vi "SubPanel_DataCollection_Rev11_v17.vi"(0 "DCPowerInformationClusterArray_Input":T8(array[cluster]), 1 "VISAPowerInfoInputArray":T5(array[cluster]), 2 "Run Data SubPanel Input":T4, 3 "RF Block Input Array":T3[](array[typedef]), 4 "Oscilloscope Info Array":T7(array[cluster]) {"vertical coupling" items=["AC", "DC", "Ground"]}, 5 "Plot Color Array":u32[](array[colorbox])=[16711686, 65351, 8978420, 14474240, 16139007, 16752640, 8958719, 16758973, 16777215, 46792, 11992992, 12961221, 16763690, 12600063, 16711835, 2953983, 40796, 13111296, 13352613, 9221011, 12964076, 12819897, 65442, 16776704, 14540253, 16740729, 10658047, 10813344, 16753521, 13413843, 8691115, 10339240, 14401205, 16746704, 7467519, 16775978, 13872558, 11387603, 13354405, 10420227, 13107364, 4060, 35208, 11817216, 7566080, 40796, 7539456, 2837073, 6372186, 7499083, 10648702, 16757152], 6 "New Run?":bool, 7 "error in":errorcluster) -> (20 "DCPowerInformationClusterArray_Output":T8(array[cluster]), 21 "VISAPowerInfoInputOutput":T5(array[cluster]), 22 "Run Data SubPanel Output":T4, 23 "RF Subpanel Output":T3[](array[typedef]), 24 "Oscilloscope Info Array":T7(array[cluster]) {"vertical coupling" items=["AC", "DC", "Ground"]}, 25 "Reinitialize?":bool, 26 "Data Was Collected?":bool, 27 "error out":errorcluster)   [LabVIEW 2019]
uses:
  Controls/DataBlockControl.ctl
  <instrlib>/niScope/Controls/niScope vertical coupling.ctl
  Controls/RFBlockControl.ctl
  Controls/QueueDataControl_V3.ctl
  <instrlib>/niScope/Acquire/Fetch/niScope Multi Fetch Binary 16.vi
  <vilib>/Utility/file.llb/Write Delimited Spreadsheet (string).vi
panel:
  in  "stop":bool
  out "wfm 2":i16[][][](array[numeric])
  out "Array":i32[](array[numeric])
  out "wfm":i16[][](array[numeric])
  in  "Total Time X Min":dbl
  in  "Total Time X Max":dbl
  in  "Total Current Y Min":dbl
  in  "Total Current Y Max":dbl
  in  "Total Voltage Y Min":dbl
  in  "Total Voltage Y Max":dbl
  in  "Total Measurement Range Update":bool
  in  "Device Powered?":bool=TRUE
  out "output cluster":T2 {"vertical coupling" items=["AC", "DC", "Ground"]}
  in  "Live Measurement Range Update":bool
  in  "Live Current Y Min":dbl
  in  "Live Current Y Max":dbl
  in  "Live Voltage Y Min":dbl
  in  "Live Voltage Y Max":dbl
  out "Current Measurements Live":cluster{dbl[], dbl[]}[](graph)
  out "Voltage Measurements Live":cluster{dbl[], dbl[]}[](graph)
  out "Voltage Waveform Array":waveform(dbl)[](graph)
  out "Current Waveform Array":waveform(dbl)[](graph)
  out "Current Measurements Total":cluster{dbl[], dbl[]}[](graph)
  out "Voltage Measurements Total":cluster{dbl[], dbl[]}[](graph)
  out "Exiting":bool
  out "Full Run Information":string
  out "Ready For Next Run?":bool
  in  "Next Run":bool
  out "Recording Data":bool
  in  "Record Data Toggle":bool
  out "error of collection":errorcluster
  in  "force exit SubVI":bool
  out "RF Block Parameters Output":T3
  in  "Oscilloscope Info Array":T6(array[cluster]) {"vertical coupling" items=["AC", "DC", "Ground"]}
  out "seconds since 1Jan1904 2":timestamp
  out "seconds since 1Jan1904":timestamp
  out "Numeric 2":i32
  out "Numeric":i32
  out "RFSourceInfoArray":string[][](array[string])
  out "OscilloscopeInfoArray":string[][](array[string])
  out "DCPowerInfoArray":string[][](array[string])
  # "Background information (Important)\nThere are three sets of voltage/current graphs\n\nOne is live always and just shows what all the channels look like _______ Waveform Array\n\nOne is live when measuring and shows some duration of the recording _______ Measurements Live\n\nOne shows the entire duration of the run, but it will take a few seconds to compile, just be patient it will populate\n\n\nInstructions (More Important)"
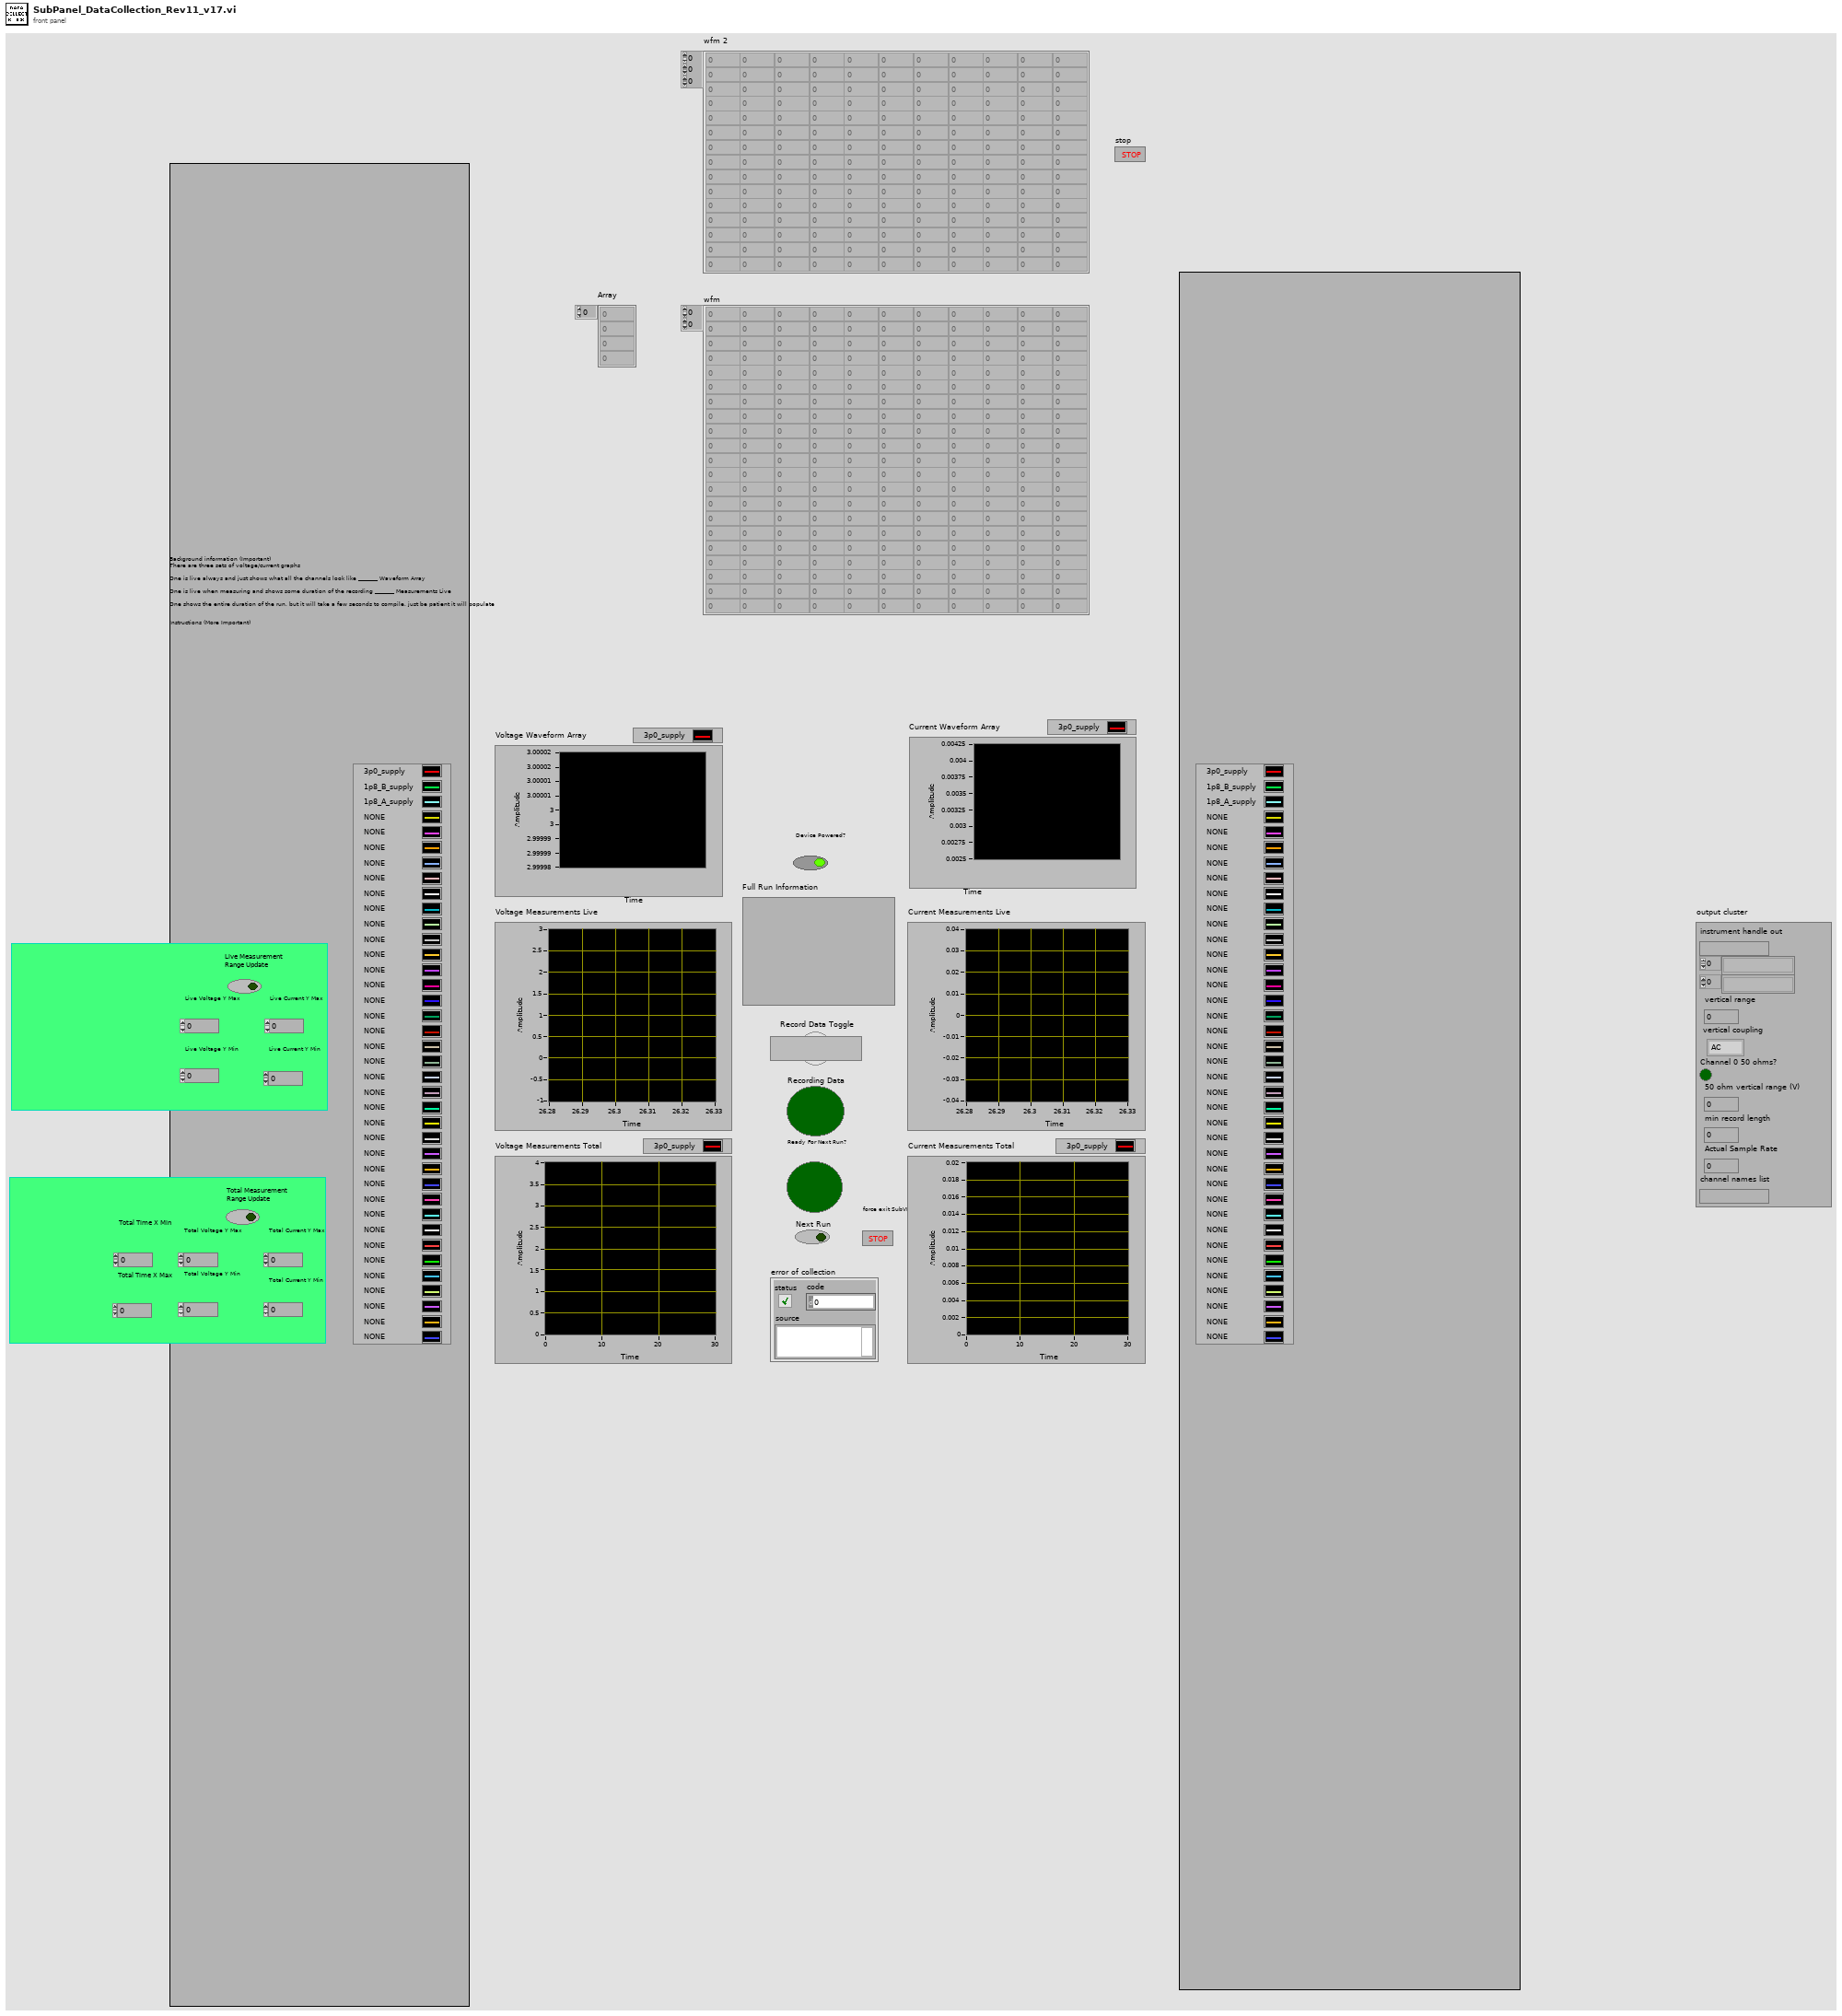
[diagram p1: front panel]
types:
  T1 = typedef "niScope vertical coupling.ctl" = i32
  T2 = cluster{"instrument handle out":refnum<k15>, string[], string[], "vertical range":dbl, "vertical coupling":T1, "Channel 0 50 ohms?":bool, "50 ohm vertical range (V)":dbl, "min record length":i32, "Actual Sample Rate":dbl, "channel names list":string}
  T3 = typedef "RFBlockControl.ctl" = cluster{"VISA resource name":refnum<visa-resource-name>, "RF Power State In":bool, "Frequency (GHz) Output":dbl, "Power (dBm) Output":dbl, "Instrument Name":string}
  T4 = typedef "DataBlockControl.ctl" = cluster{"Run Folder Parent Directory":path, "DUT":string, "Ion (ex Kr)":string, "Board Number":string, "Effective LET":string, "Test Type":enum16{"Single Event Latchup", "Single Event Transient", "Single Event Upset"}}
  T5 = cluster{"VISA resource name":refnum<visa-resource-name>, "String List":string, string[], "Input Array (Voltage,Current_Limit)":dbl[], "Input Array (Voltage,Current_Limit)":dbl[], "Channel Names":string[], "read buffer":string}[]
  T6 = cluster{"instrument handle out":refnum<k15>, "channel numbers array":string[], "channel names array":string[], "vertical range":dbl, "vertical coupling":T1, "Channel 0 50 ohms?":bool, "50 ohm vertical range (V)":dbl, "min record length":i32, "Actual Sample Rate":dbl}[]
  T7 = cluster{"instrument handle out":refnum<k15>, string[], string[], "vertical range":dbl, "vertical coupling":T1, "Channel 0 50 ohms?":bool, "50 ohm vertical range (V)":dbl, "min record length":i32, "Actual Sample Rate":dbl, "channel names list":string}[]
  T8 = cluster{"IVI Refnum out":refnum<k15>, "Active Channel Numbers String List":string, "Active Channel Numbers Array":string[], "Active Channel Voltage Array":dbl[], "Active Channel Names Array":string[], "Active Channel Current Limit Array":dbl[], "Active Channel Measure Record Delta Time Array":dbl[], "All Channel Numbers Array":string[]}[]
  T9 = typedef "QueueDataControl_V3.ctl" = cluster{"Array of fetched data":dbl[][][], "Channel Names Array":string[], "Voltage Waveform Array":waveform(dbl)[], "Current Waveform Array":waveform(dbl)[], "Resetting Time":timestamp}
  T10 = cluster{"IVI Refnum out":refnum<k15>, string, "voltage level channel 23":dbl, "Channel Name 23":string, "Current Limit":dbl, "Measure Record dt":dbl, string}[]
  T11 = cluster{timestamp[], "wfm info":cluster{"actualSamples":i32, "absoluteInitialX":dbl, "relativeInitialX":dbl, "xIncrement":dbl, "offset":dbl, "gain":dbl, "reserved1":dbl, "reserved2":dbl}[][], "wfm":i16[][][]}
  T12 = cluster{"actualSamples":i32, "absoluteInitialX":dbl, "relativeInitialX":dbl, "xIncrement":dbl, "offset":dbl, "gain":dbl, "reserved1":dbl, "reserved2":dbl}[]
  T13 = cluster{"created path":path, "DCPowerInformation_byChannel":cluster{"IVI Refnum out":refnum<k15>, string, "voltage level channel 23":dbl, "Channel Name 23":string, "Current Limit":dbl, "Measure Record dt":dbl, string}[], string[]}
  T14 = cluster{"Array of fetched data":dbl[][], string, i32[]}
  T15 = enum16{"open", "replace", "create", "open or create", "replace or create", "replace or create with confirmation"}
  T16 = enum16{"Single Event Latchup", "Single Event Transient", "Single Event Upset"}
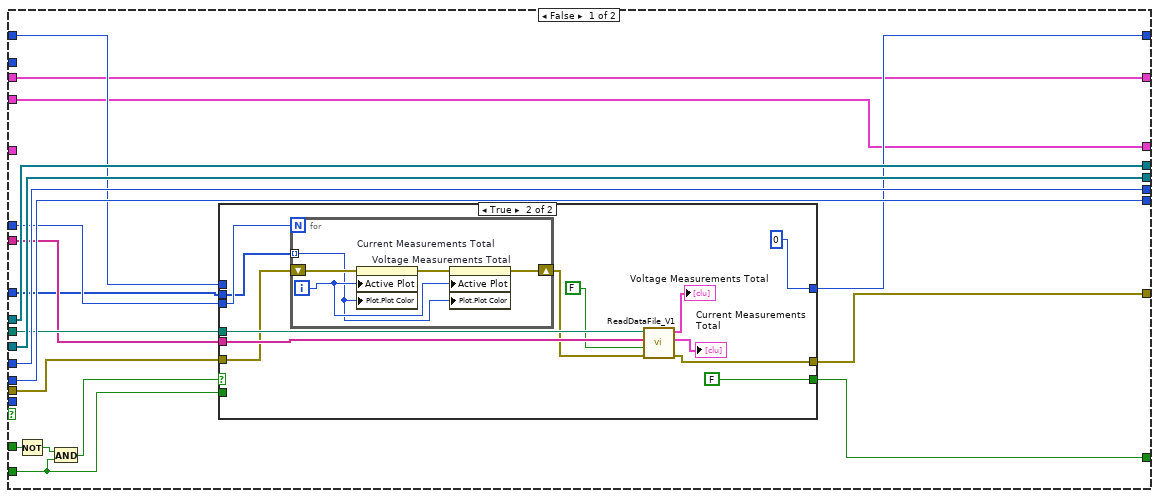
[diagram p7: hidden frame]
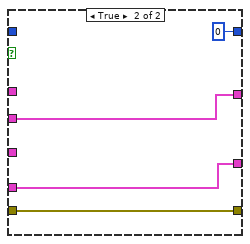
[diagram p9: hidden frame]
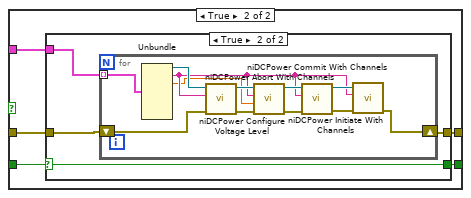
[diagram p10: hidden frame]
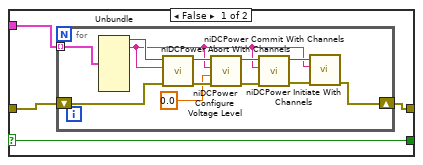
[diagram p11: hidden frame]
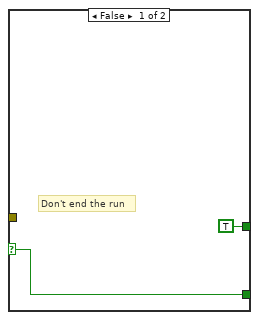
[diagram p12: hidden frame]
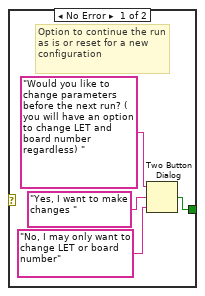
[diagram p13: hidden frame]
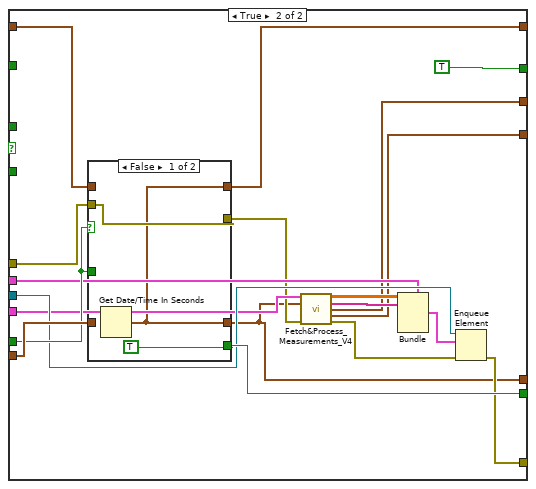
[diagram p16: hidden frame]
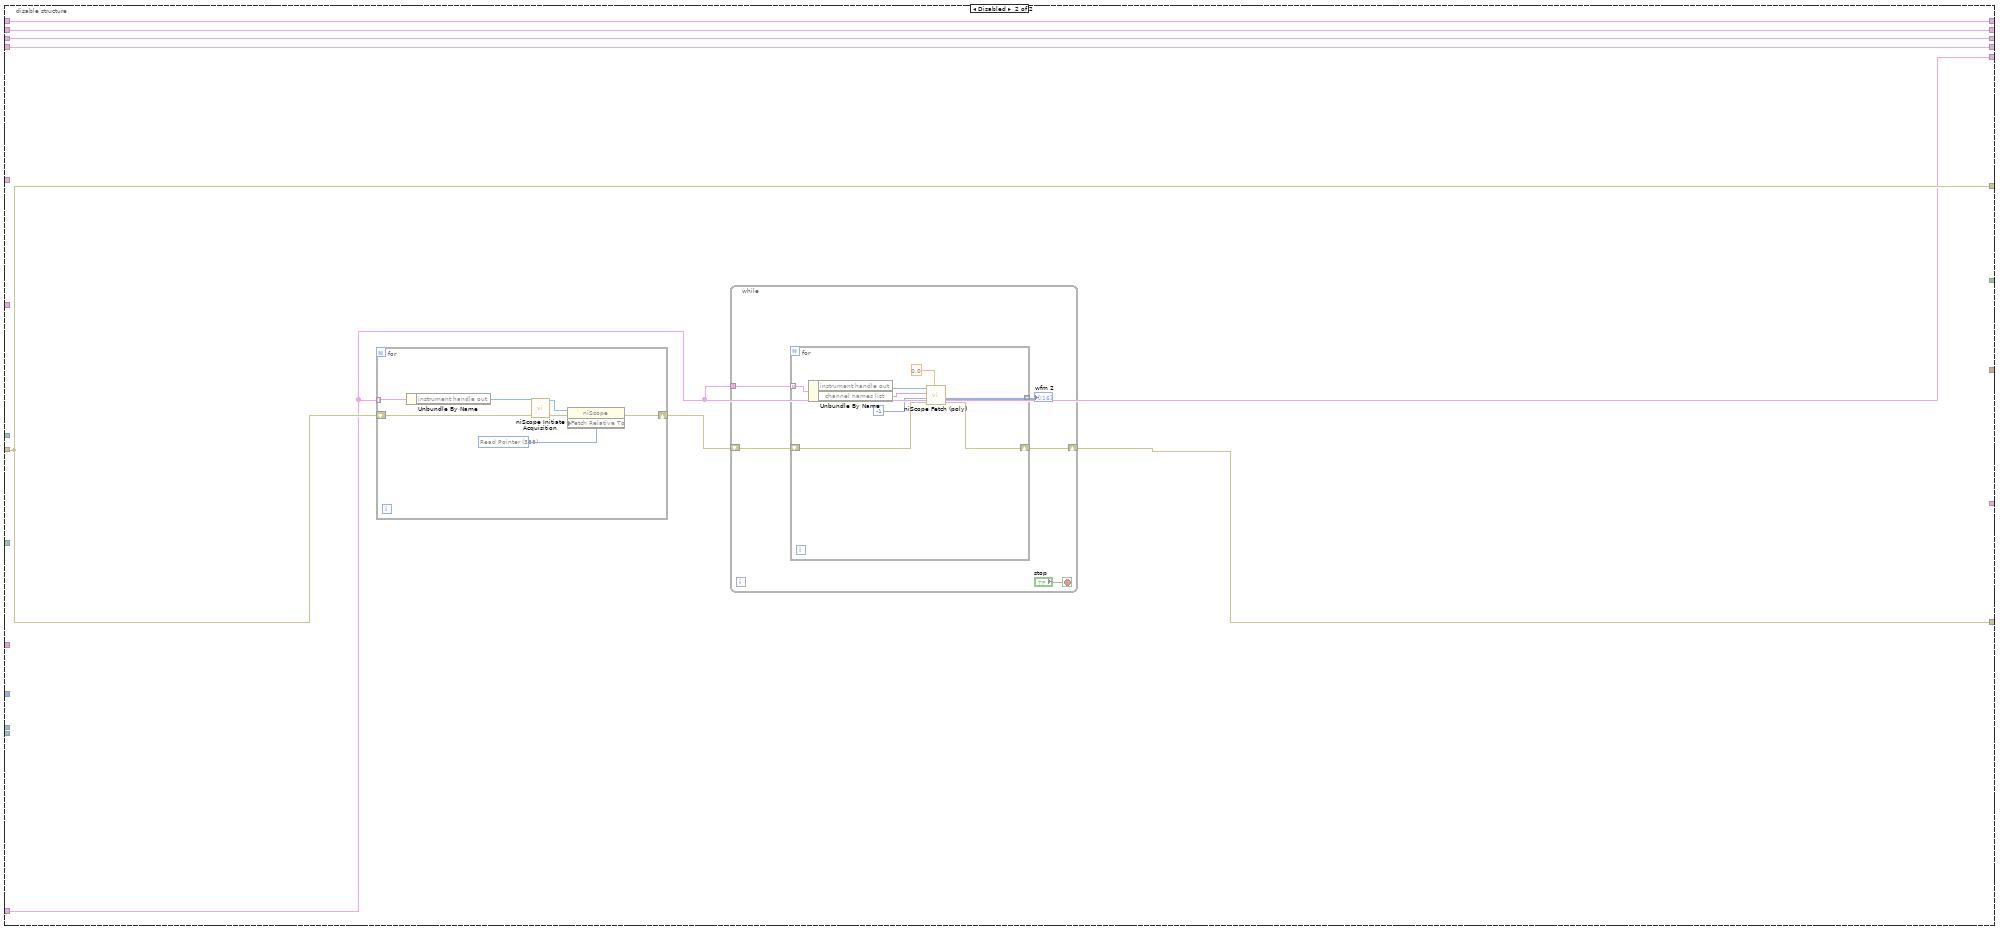
[diagram p18: hidden frame]
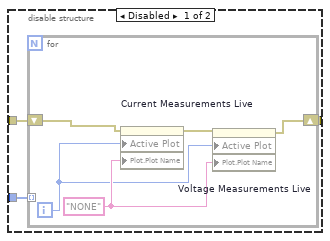
[diagram p19: hidden frame]
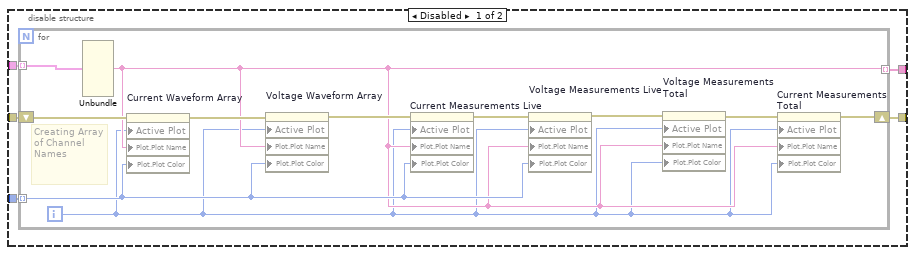
[diagram p20: hidden frame]
diagram:
  (unwired) string[] ["Instrument Name", "Channel Name", "Instrument Channel Number", "Voltage (V)", "Current Limit (A)", "Measure Record delta Time (s)"] ("new element/subarray")
  w41 = T9 {"Array of fetched data"=[], "Channel Names Array"=[], "Voltage Waveform Array"=[], "Current Waveform Array"=[], "Resetting Time"=timestamp(0 s since 1904-01-01)} ("DCPower Queue Data Double Array Format")
  (unwired) T9 {"Array of fetched data"=[], "Channel Names Array"=[], "Voltage Waveform Array"=[], "Current Waveform Array"=[], "Resetting Time"=timestamp(0 s since 1904-01-01)} ("DCPower Double Array Queue")
  (unwired) T4 {"Run Folder Parent Directory"=path "", "DUT"="", "Ion (ex Kr)"="", "Board Number"="", "Effective LET"="", "Test Type"=enum."Single Event Latchup"} ("Run Data Configuration")
  # "Initiating the queue"
  # "echoing run information"
  # "Checking if this is a new run. If it is, a new folder is created along with references to a datafile node. If it is not new (i.e. you didn't start recording data because you needed to make a last minute change and pressed forced exit subvi), the previous folder that is theoretically empty (or just has the .txt files is used"
  # "If yes, you go into this subVI"
  # "This is the message at the beginning confirming if you want to make small changes to the program (i.e. LET)"
  # "Parameters from the configuration stage of this program"
  # "Need to change to reflect number of channels that are being recorded. Collect this from a parameters file eventually that will be created"
  # "Initiating all of the DC Power instruments (doing this here so because we force abort channels in the DCPower setup because buffer overflow issues. Iterating over the instrument array and the active channel list"
  n1 = flat-sequence {
    tunnel: [w74] -> w55
    tunnel: "error in" -> [w64]
    tunnel: [w78] -> w59
    tunnel: "Run Data SubPanel Input" -> [w66]
    frame #0 {
      n2 = disable-structure shown="Enabled" {
        disable-tunnel: w64 -> [w81 w92]
        disable-tunnel: [w90 w92] -> w63
        frame Enabled {
          n3 = property on="Voltage Measurements Live" class="XYGraph (strict)"(error in=w81, "BG Color"=u32 0 ("Plot.Plot Color"), "Plot.Plot Interpolation"=u8 2) -> (error out=w80:errorcluster)  [unwired: 1 in, 1 out]
          n4 = property on="Current Measurements Live" class="XYGraph (strict)"(error in=w80, "BG Color"=u32 0 ("Plot.Plot Color"), "Plot.Plot Interpolation"=u8 2) -> (error out=w79:errorcluster)  [unwired: 1 in, 1 out]
          n5 = property on="Voltage Measurements Total" class="XYGraph (strict)"(error in=w79, "BG Color"=u32 0 ("Plot.Plot Color"), "Plot.Plot Interpolation"=u8 2) -> (error out=w91:errorcluster)  [unwired: 1 in, 1 out]
          n6 = property on="Current Measurements Total" class="XYGraph (strict)"(error in=w91, "BG Color"=u32 0 ("Plot.Plot Color"), "Plot.Plot Interpolation"=u8 2) -> (error out=w90:errorcluster)  [unwired: 1 in, 1 out]
        }
        frame Disabled {
        }
      }
      n7 = local write "Voltage Measurements Total"(cluster{dbl[], dbl[]}[] [] ("Voltage Measurements")) -> ()
      n8 = local write "Current Measurements Total"(cluster{dbl[], dbl[]}[] [] ("Current Measurements")) -> ()
      n9 = local write "Recording Data"(FALSE ("Recording Data")) -> ()
      n10 = local write "Exiting"(FALSE ("Forced Exit")) -> ()
      n11 = call "Convert_RunInfoCluster_2_RunInfoStringList.vi"("error in"=w63, "Run Number"="", "Run Data SubPanel Input"=w66) -> ("error output"=w67:errorcluster, "Run Data Output"=w68:string)
      n12 = call "Display Message to User"("error in (no error)"=w67, "Enable"=TRUE, "Message"=w68) -> ("error out"=w74:errorcluster)  [unwired: 7 in, 1 out]
      n13 = Two Button Dialog(message="Changing the LET?", 1:"No" ("F button name (\"Cancel\")"), 2:"Yes" ("T button name (\"OK\")")) -> (T button?=w78:bool)
    }
  }
  n14 = call "Convert_InstrumentReferenceArray_2_ChannelReferenceArray.vi"("error in (no error)"=w55, "DCPowerInformationClusterArray_Input"="DCPowerInformationClusterArray_Input") -> ("error out"=w54:errorcluster, "DCPowerInformation_byChannel"=w1:T10)
  n15 = case shown="True" w59 {
    tunnel: "Run Data SubPanel Input" -> [w94 w98]
    tunnel: [w94 w97] -> w25
    tunnel: [w93 w96] -> w56
    tunnel: w54 -> [w93 w95]
    frame False {
    }
    frame True {
      n16 = disable-structure shown="Enabled" {
        disable-tunnel: w98 -> [w102 w104]
        disable-tunnel: [w101 w103] -> w97
        disable-tunnel: [w100 w106] -> w96
        disable-tunnel: w95 -> [w99 w105]
        frame Disabled {
          n17 = call "Change_RunInfo.vi"("error in (no error)"=w99, "Run Data SubPanel in"=w102) -> ("error out"=w100:errorcluster, "Run Data SubPanel out"=w101:T4)
        }
        frame Enabled {
          n18 = call "Change_RunInfo_V2.vi"("error in (no error)"=w105, "Run Data SubPanel in"=w104) -> ("error out"=w106:errorcluster, "Run Data SubPanel out"=w103:T4)
        }
      }
    }
  }
  n19 = Unbundle(w25) -> ("Run Folder Parent Directory"=w57:path)  [unwired: 5 out]
  n20 = List Folder(path=w57, error in=w56) -> (folder names=w58:string[], error out=w44:errorcluster)  [unwired: 2 in, 2 out]
  n21 = Array Size(array=w58) -> (size(s)=w47:i32)
  n22 = case shown="True" "New Run?" {
    selector: "New Run?" -> [w108 w111]
    tunnel: [w109 w113] -> w48
    tunnel: w47 -> [w109 w112]
    tunnel: [w108 w111] -> w46
    tunnel: [w107 w110] -> w45
    tunnel: w44 -> [w107 w110]
    frame False {
    }
    frame True {
      n23 = Increment(x=w112) -> (x+1=w113:i32)
    }
  }
  n24 = Number To Decimal String(number=w48) -> (decimal integer string=w51:string)  [unwired: 1 in]
  n25 = Concatenate Strings("Run_", w51) -> (w24:string)
  n26 = Array Size(array=w1) -> (size(s)=w43:i32)
  n27 = call "InitialFileFolderCreation_V2.vi"("New Run?"=w46, "error in (no error)"=w45, "Run Number"=w24, "DCPowerArrayClusterSize"=w43, "base path"=w57) -> ("error out"=w23:errorcluster, "SupplementalDataFileReferenceObjectArray"=w52:refnum<file>[], "DataFileReferenceObjectArray"=w53:refnum<file>[], "created path"=w27:path)  [unwired: 3 in]
  n28 = call "Convert_RunInfoCluster_2_RunInfoStringList.vi"("error in"=w23, "Run Number"=w24, "Run Data SubPanel Input"=w25) -> ("error output"=w22:errorcluster, "Run Data Output"=→"Full Run Information":string)
  n29 = for {
    shift-right: [w114] -> w15
    shift-left: w22 -> [w116]
    tunnel: "DCPowerInformationClusterArray_Input" -> [w118] mode=indexing
    n30 = Unbundle(w118) -> ("IVI Refnum out"=w115:refnum<k15>, "Active Channel Numbers String List"=w117:string)  [unwired: 6 out]
    n31 = call <instrlib>:"niDCPower Initiate With Channels.vi"("error in (no error)"=w116, "channel name"=w117, "instrument handle"=w115) -> ("error out"=w114:errorcluster)  [unwired: 7 in, 1 out]
  }
  n32 = disable-structure shown="Enabled" {
    disable-tunnel: "Plot Color Array" -> [w121 _]
    disable-tunnel: [w120 w127] -> w16
    disable-tunnel: w15 -> [w119 w127]
    frame Disabled {
      n33 = for {
        shift-right: [w124] -> w120
        shift-left: w119 -> [w126]
        tunnel: w121 -> [_] mode=indexing
        i -> [w122]
        w123 = "NONE" ("Plot.Plot Name")
        n34 = property on="Current Measurements Live" class="XYGraph (strict)"(error in=w126, "Active Plot"=w122, "Plot.Plot Name"=w123) -> (error out=w125:errorcluster)  [unwired: 1 in, 1 out]
        n35 = property on="Voltage Measurements Live" class="XYGraph (strict)"(error in=w125, "Active Plot"=w122, "Plot.Plot Name"=w123) -> (error out=w124:errorcluster)  [unwired: 1 in, 1 out]
      }
    }
    frame Enabled {
    }
  }
  n36 = case shown="Error .." w16 {
    selector: w16 -> [w128 _]
    tunnel: [w128 w129] -> w4
    tunnel: w15 -> [_ w129]
    frame No Error {
    }
    frame Error {
    }
  }
  n37 = disable-structure shown="Enabled" {
    disable-tunnel: [w134 w147] -> w18
    disable-tunnel: w1 -> [w133 w148]
    disable-tunnel: "Plot Color Array" -> [w132 _]
    disable-tunnel: [w131 w146] -> w5
    disable-tunnel: w4 -> [w130 w146]
    frame Disabled {
      n38 = for {
        tunnel: w133 -> [w144] mode=indexing
        tunnel: [w136] -> w134 mode=indexing
        shift-right: [w137] -> w131
        shift-left: w130 -> [w141]
        tunnel: w132 -> [w140] mode=indexing
        i -> [w135]
        # "Creating Array of Channel Names"
        n39 = Unbundle(w144) -> ("Channel Name 23"=w136:string)  [unwired: 6 out]
        n40 = property on="Current Waveform Array" class="WFChart (strict)"(error in=w141, "Active Plot"=w135, "Plot.Plot Name"=w136, "Plot.Plot Color"=w140) -> (error out=w143:errorcluster)  [unwired: 1 in, 1 out]
        n41 = property on="Voltage Waveform Array" class="WFChart (strict)"(error in=w143, "Active Plot"=w135, "Plot.Plot Name"=w136, "Plot.Plot Color"=w140) -> (error out=w142:errorcluster)  [unwired: 1 in, 1 out]
        n42 = property on="Current Measurements Live" class="XYGraph (strict)"(error in=w142, "Active Plot"=w135, "Plot.Plot Name"=w136, "Plot.Plot Color"=w140) -> (error out=w145:errorcluster)  [unwired: 1 in, 1 out]
        n43 = property on="Voltage Measurements Live" class="XYGraph (strict)"(error in=w145, "Active Plot"=w135, "Plot.Plot Name"=w136, "Plot.Plot Color"=w140) -> (error out=w139:errorcluster)  [unwired: 1 in, 1 out]
        n44 = property on="Voltage Measurements Total" class="XYGraph (strict)"(error in=w139, "Active Plot"=w135, "Plot.Plot Name"=w136, "Plot.Plot Color"=w135) -> (error out=w138:errorcluster)  [unwired: 1 in, 1 out]
        n45 = property on="Current Measurements Total" class="XYGraph (strict)"(error in=w138, "Active Plot"=w135, "Plot.Plot Name"=w136, "Plot.Plot Color"=w135) -> (error out=w137:errorcluster)  [unwired: 1 in, 1 out]
      }
    }
    frame Enabled {
      n46 = for {
        tunnel: w148 -> [w150] mode=indexing
        tunnel: [w149] -> w147 mode=indexing
        n47 = Unbundle(w150) -> ("Channel Name 23"=w149:string)  [unwired: 6 out]
      }
    }
  }
  n48 = case shown="Error .." w5 {
    selector: w5 -> [w151 _]
    tunnel: [w151 w152] -> w3
    tunnel: w4 -> [_ w152]
    frame No Error {
    }
    frame Error {
    }
  }
  n49 = disable-structure shown="Enabled" {
    disable-tunnel: w3 -> [w156 w158]
    disable-tunnel: [w155 w158] -> w8
    disable-tunnel: [w154 _] -> w19
    disable-tunnel: w41 -> [w153 _]
    frame Enabled {
      n50 = Obtain Queue(name (unnamed)="DCPowerQueue", element data type=w153, error in (no error)=w156) -> (queue out=w154:refnum<queue>, error out=w155:errorcluster)  [unwired: 2 in, 1 out]
    }
    frame Disabled {
    }
  }
  n51 = disable-structure shown="Enabled" {
    disable-tunnel: "VISAPowerInfoInputArray" -> [w201 w618]
    disable-tunnel: w53 -> [w197 _]
    disable-tunnel: w52 -> [w196 _]
    disable-tunnel: [w193 w615] -> w42
    disable-tunnel: w41 -> [w192 _]
    disable-tunnel: [w189 w612] -> w40
    disable-tunnel: [w186 _] -> w38
    disable-tunnel: [w185 w616] -> w36
    disable-tunnel: [w184 w617] -> w34
    disable-tunnel: [w183 w618] -> w32
    disable-tunnel: [w182 w619] -> w31
    disable-tunnel: [w181 _] -> w30
    disable-tunnel: w27 -> [w180 _]
    disable-tunnel: w25 -> [w178 w617]
    disable-tunnel: "RF Block Input Array" -> [w175 w616]
    disable-tunnel: w19 -> [w171 _]
    disable-tunnel: w18 -> [w170 _]
    disable-tunnel: w1 -> [w169 _]
    disable-tunnel: "Plot Color Array" -> [w168 _]
    disable-tunnel: [w167 _] -> w12
    disable-tunnel: "Oscilloscope Info Array" -> [w166 w613]
    disable-tunnel: w8 -> [w162 w615]
    disable-tunnel: "DCPowerInformationClusterArray_Input" -> [w161 w619]
    disable-tunnel: [w159 w613] -> w2
    frame Enabled {
      w174 = cluster{dbl[], dbl[]}[] [] ("array")
      (unwired) 10000 ("binary file indexor in")
      # "A flag to state if the devices are powered on or off"
      # "Need to make a function that will decrease the amount of loops if there are more channels active. Just exponential decay or a X/Y function but need some kind of offset which will probably be experimentally determined"
      # "Reset the graph that is saving every 10 seconds of data. Every reset the low bound of the ten seconds is"
      # "Indicator if the system is ready for another run. Also indicates if data was actually collected"
      # "Resets the system to start recording"
      # "A flag to ensure the warning message shows only once and doesn't lock the system"
      n52 = disable-structure shown="Enabled" {
        disable-tunnel: w166 -> [w209 w265]
        disable-tunnel: [w206 w266] -> w165
        disable-tunnel: w162 -> [w210 w266]
        disable-tunnel: [w203 w265] -> w159
        frame Enabled {
          w212 = T11 {[], "wfm info"=[], "wfm"=[]} ("output cluster")
          n53 = for {
            tunnel: w209 -> [w226] mode=indexing
            shift-right: [w223] -> w211
            shift-left: w210 -> [w227]
            tunnel: [w220] -> w204 mode=indexing
            w221 = 388 items=["Start"=482, "Trigger"=483, "Pretrigger"=477, "Now"=481, "Read Pointer"=388] ("Fetch:Fetch Relative To")
            n54 = Unbundle By Name(w226) -> ("instrument handle out"=w225:refnum<k15>)
            n55 = call <instrlib>:"niScope Initiate Acquisition.vi"("instrument handle"=w225, "error in"=w227) -> ("instrument handle out"=w224:refnum<k15>, "error out"=w222:errorcluster)  [unwired: 12 in]
            n56 = property class="niScope"(reference=w224, error in=w222, "Fetch Relative To"=w221) -> (error out=w223:errorcluster, "Binary Sample Width"=w220:i32)  [unwired: 1 out]
          }
          "Array" <- w204
          n57 = Obtain Queue(name (unnamed)="OscilloscopeDataQueue", element data type=w212, error in (no error)=w211) -> (queue out=w213:refnum<queue>, error out=w215:errorcluster)  [unwired: 2 in, 1 out]
          n58 = while {
            shift-right: [w236] -> w207
            shift-left: w215 -> [w239]
            shift-right: [w237] -> w205
            shift-left: w209 -> [w237]
            tunnel: w213 -> [_]
            tunnel: w212 -> [w238]
            tunnel: [w235] -> _
            shift-right: [w229] -> _
            shift-left: FALSE ("x") -> [w230]
            i -> [w228]
            stop <- w234 stop-if-true
            # "BASE OFF OF TAMU POWER SCRIPTS"
            n59 = for {
              tunnel: w237 -> [w245] mode=indexing
              shift-right: [w253] -> w236
              shift-left: w239 -> [w249]
              tunnel: [w252] -> w232 mode=indexing
              tunnel: [w251] -> w231 mode=indexing
              tunnel: [w240] -> w233 mode=indexing
              shift-right: [w246] -> w229
              shift-left: w230 -> [w243]
              tunnel: w228 -> [w244]
              tunnel: w228 -> [w241]
              i -> [w250]
              n60 = Get Date/Time In Seconds() -> (seconds since 1Jan1904=w240:timestamp)
              n61 = Not(x=w243) -> (.not. x?=w248:bool)
              n62 = Unbundle By Name(w245) -> ("instrument handle out"=w257:refnum<k15>, "channel names list"=w255:string)
              n63 = And(x=w249, y=w248) -> (x .and. y?=w247:bool)
              n64 = Equal To 0?(x=w241) -> (x = 0?=w242:bool)
              n65 = case shown="True" w247 {
                tunnel: w250 -> [_ w264]
                tunnel: [w259 TRUE] -> w246
                tunnel: w245 -> [_ w263]
                tunnel: w244 -> [_ w262]
                tunnel: w243 -> [w259 _]
                tunnel: w240 -> [_ w260]
                frame False {
                }
                frame True {
                  "Numeric" <- w264
                  "output cluster" <- w263
                  "Numeric 2" <- w262
                  "seconds since 1Jan1904" <- w260
                }
              }
              n66 = case shown="True" w242 {
                tunnel: w240 -> [_ w258]
                frame False {
                }
                frame True {
                  "seconds since 1Jan1904 2" <- w258
                }
              }
              n67 = call-poly <instrlib>:"niScope Fetch (poly).vi"("timeout"=0.0, "error in"=w249, "numSamples"=-1, "channels"=w255, "instrument handle"=w257) -> ("error out"=w253:errorcluster, "wfm"=w251:i16[][], "wfm info"=w252:T12)  [unwired: 3 in, 1 out]
              "wfm" <- w251
            }
            n68 = Bundle(cluster=w238, w233, "wfm info"=w232, "wfm"=w231) -> (w235:T11)
            n69 = local read "Exiting"() -> (w234:bool)
          }
          n70 = for {
            shift-right: [w218] -> w206
            shift-left: w207 -> [w219]
            tunnel: w205 -> [w216] mode=indexing
            tunnel: [w216] -> w203 mode=indexing
            n71 = Unbundle By Name(w216) -> ("instrument handle out"=w217:refnum<k15>)
            n72 = call <instrlib>:"niScope Abort.vi"("instrument handle"=w217, "error in"=w219) -> ("error out"=w218:errorcluster)  [unwired: 12 in, 1 out]
          }
        }
        frame Disabled {
          # "get the 1355 board"
        }
      }
      n73 = Bundle("created path"=w180, "DCPowerInformation_byChannel"=w169, w170) -> (w186:T13)  [unwired: 1 in]
      n74 = Array Size(array=w170) -> (size(s)=w173:i32)
      n75 = Get Date/Time In Seconds() -> (seconds since 1Jan1904=w179:timestamp)
      n76 = while {
        shift-right: [w504] -> w182
        shift-left: w161 -> [w504]
        shift-right: [w507] -> w183
        shift-left: w201 -> [w507]
        shift-right: [w506] -> w184
        shift-left: w178 -> [w506]
        shift-right: [w505] -> w185
        shift-left: w175 -> [w505]
        shift-right: [w476] -> w193
        shift-left: w162 -> [w503]
        tunnel: w169 -> [w473]
        shift-right: [w502] -> _
        shift-left: FALSE -> [w499]
        tunnel: w171 -> [w501]
        shift-right: [w486] -> _
        shift-left: FALSE -> [w491]
        tunnel: [w495] -> w200
        shift-right: [w489] -> _
        shift-left: TRUE ("x .and. y?") -> [w490]
        shift-right: [w487] -> _
        shift-left: w179 -> [w488]
        tunnel: [w486] -> w181
        tunnel: w192 -> [w484]
        shift-right: [w481] -> w167
        shift-left: timestamp(0 s since 1904-01-01) ("seconds since 1Jan1904") -> [w480]
        shift-right: [w470] -> _
        shift-left: TRUE -> [w469]
        stop <- w485 stop-if-true
        # "If I am going to reset the entire configuration or if we are going up in LET only. True, reset the system. False, don't reset the system"
        n77 = Not(x=w491) -> (.not. x?=w493:bool)
        n78 = And(x="Record Data Toggle", y=w493) -> (x .and. y?=w494:bool)
        "Recording Data" <- w494
        n79 = case shown="False" w494 {
          tunnel: w473 -> [w575 w590]
          tunnel: w503 -> [w573 w597]
          tunnel: [w563 w585] -> w483
          tunnel: [w564 w584] -> w482
          tunnel: w499 -> [_ w595]
          tunnel: [FALSE w596] -> w502
          tunnel: w501 -> [_ w594]
          tunnel: [w562 w593] -> w475
          tunnel: "Record Data Toggle" -> [w570 _]
          tunnel: w491 -> [w571 _]
          tunnel: w490 -> [w566 _]
          tunnel: [w567 TRUE] -> w489
          tunnel: w488 -> [w565 w598]
          tunnel: [w565 w588] -> w487
          tunnel: w484 -> [_ w592]
          tunnel: [w561 w582] -> w481
          tunnel: w480 -> [w561 w581]
          frame False {
            n80 = And(x=w570, y=w571) -> (x .and. y?=w569:bool)
            n81 = And(x=w566, y=w569) -> (x .and. y?=w568:bool)
            n82 = case shown="True" w568 {
              tunnel: [w577 w579] -> w572
              tunnel: w573 -> [w577 w580]
              tunnel: [w576 FALSE] -> w567
              tunnel: w566 -> [w576 _]
              frame False {
              }
              frame True {
                n83 = call "Display Message to User2"("error in (no error)"=w580) -> ("error out"=w579:errorcluster)  [unwired: 9 in, 1 out]
              }
            }
            n84 = call "Fetch&Process_Measurements_V4.vi"("DCPowerInformation_byChannel"=w575, "Initial Time"=w565, "error in (no error)"=w572) -> ("Current Waveform Array"=w563:waveform(dbl)[], "Voltage Waveform Array"=w564:waveform(dbl)[], "error out"=w562:errorcluster)  [unwired: 6 in, 4 out]
          }
          frame True {
            n85 = case shown="False" w595 {
              tunnel: [w600 w606] -> w588
              tunnel: w598 -> [_ w606]
              tunnel: w597 -> [w601 w605]
              tunnel: [w601 w605] -> w589
              tunnel: [TRUE w604] -> w596
              tunnel: w595 -> [_ w604]
              tunnel: [w600 w603] -> w582
              tunnel: w581 -> [_ w603]
              frame False {
                n86 = Get Date/Time In Seconds() -> (seconds since 1Jan1904=w600:timestamp)
              }
              frame True {
              }
            }
            n87 = call "Fetch&Process_Measurements_V4.vi"("DCPowerInformation_byChannel"=w590, "Initial Time"=w588, "error in (no error)"=w589) -> ("Data As dbl Array"=w587:dbl[][][], "Channel Number Array"=w586:string[], "Current Waveform Array"=w585:waveform(dbl)[], "Voltage Waveform Array"=w584:waveform(dbl)[], "error out"=w583:errorcluster)  [unwired: 6 in, 2 out]
            n88 = Bundle(cluster=w592, "Array of fetched data"=w587, "Channel Names Array"=w586) -> (w591:T9)  [unwired: 3 in]
            n89 = Enqueue Element(queue=w594, element=w591, error in (no error)=w583) -> (error out=w593:errorcluster)  [unwired: 1 in, 2 out]
          }
        }
        "Current Waveform Array" <- w483
        "Voltage Waveform Array" <- w482
        n90 = Not(x=w494) -> (.not. x?=w500:bool)
        n91 = And(x=w500, y=w499) -> (x .and. y?=w498:bool)
        n92 = Exclusive Or(1:"Device Powered?", 2:w469) -> (0:w472:bool)
        n93 = case shown="False" w472 {
          tunnel: [w509 w513] -> w474
          tunnel: w475 -> [w509 w512]
          tunnel: w473 -> [_ w514]
          tunnel: "Device Powered?" -> [w508 w511]
          tunnel: [w508 w510] -> w470
          frame False {
          }
          frame True {
            n94 = case shown="True" w511 {
              selector: w511 -> [w515 w531]
              tunnel: w514 -> [w518 w534]
              tunnel: [w516 w533] -> w513
              tunnel: w512 -> [w517 w532]
              tunnel: [w515 w531] -> w510
              frame False {
                n95 = for {
                  tunnel: w518 -> [w530] mode=indexing
                  shift-right: [w520] -> w516
                  shift-left: w517 -> [w521]
                  n96 = Unbundle(w530) -> ("IVI Refnum out"=w529:refnum<k15>, w522:string)  [unwired: 5 out]
                  n97 = call <instrlib>:"niDCPower Abort With Channels.vi"("error in (no error)"=w521, "channel name"=w522, "instrument handle"=w529) -> ("error out"=w528:errorcluster, "instrument handle out"=w527:refnum<k15>)  [unwired: 7 in]
                  n98 = call <instrlib>:"niDCPower Configure Voltage Level.vi"("error in (no error)"=w528, "voltage level"=0.0, "channel name"=w522, "instrument handle"=w527) -> ("error out"=w526:errorcluster, "instrument handle out"=w525:refnum<k15>)  [unwired: 6 in]
                  n99 = call <instrlib>:"niDCPower Commit With Channels.vi"("error in (no error)"=w526, "channel name"=w522, "instrument handle"=w525) -> ("error out"=w524:errorcluster, "instrument handle out"=w523:refnum<k15>)  [unwired: 7 in]
                  n100 = call <instrlib>:"niDCPower Initiate With Channels.vi"("error in (no error)"=w524, "channel name"=w522, "instrument handle"=w523) -> ("error out"=w520:errorcluster)  [unwired: 7 in, 1 out]
                }
              }
              frame True {
                n101 = for {
                  tunnel: w534 -> [w546] mode=indexing
                  shift-right: [w536] -> w533
                  shift-left: w532 -> [w537]
                  n102 = Unbundle(w546) -> ("IVI Refnum out"=w545:refnum<k15>, w538:string, "voltage level channel 23"=w535:dbl)  [unwired: 4 out]
                  n103 = call <instrlib>:"niDCPower Abort With Channels.vi"("error in (no error)"=w537, "channel name"=w538, "instrument handle"=w545) -> ("error out"=w544:errorcluster, "instrument handle out"=w543:refnum<k15>)  [unwired: 7 in]
                  n104 = call <instrlib>:"niDCPower Configure Voltage Level.vi"("error in (no error)"=w544, "voltage level"=w535, "channel name"=w538, "instrument handle"=w543) -> ("error out"=w542:errorcluster, "instrument handle out"=w541:refnum<k15>)  [unwired: 6 in]
                  n105 = call <instrlib>:"niDCPower Commit With Channels.vi"("error in (no error)"=w542, "channel name"=w538, "instrument handle"=w541) -> ("error out"=w540:errorcluster, "instrument handle out"=w539:refnum<k15>)  [unwired: 7 in]
                  n106 = call <instrlib>:"niDCPower Initiate With Channels.vi"("error in (no error)"=w540, "channel name"=w538, "instrument handle"=w539) -> ("error out"=w536:errorcluster)  [unwired: 7 in, 1 out]
                }
              }
            }
          }
        }
        n107 = case shown="True" w498 {
          tunnel: w474 -> [w557 w559]
          tunnel: [w558 TRUE] -> w486
          tunnel: w491 -> [w558 _]
          tunnel: [w557 w559] -> w476
          frame False {
          }
          frame True {
          }
        }
        "error of collection" <- w476
        "Ready For Next Run?" <- w486
        n108 = And(x="Next Run", y=w486) -> (x .and. y?=w497:bool)
        n109 = Or(x="force exit SubVI", y=w497) -> (x .or. y?=w478:bool)
        n110 = Or(x=w476, y=w478) -> (x .or. y?=w477:bool)
        n111 = case shown="True" w477 {
          selector: w477 -> [w548 _]
          tunnel: w476 -> [_ w551]
          tunnel: [w548 TRUE] -> w485
          tunnel: [TRUE ("T button?") w549] -> w495
          frame False {
            # "Don't end the run"
          }
          frame True {
            n112 = case shown="Error .." w551 {
              tunnel: [w552 TRUE] -> w549
              frame No Error {
                # "Option to continue the run as is or reset for a new configuration"
                n113 = Two Button Dialog(message="Would you like to change parameters before the next run? ( you will have an option to change LET and board number regardless) ", 1:"No, I may only want to change LET or board number" ("F button name (\"Cancel\")"), 2:"Yes, I want to make changes " ("T button name (\"OK\")")) -> (T button?=w552:bool)
              }
              frame Error {
                # "End the run immediately. There is an error or an immediate issue with the VI"
              }
            }
          }
        }
        "Exiting" <- w485
      }
      "Reinitialize?" <- w200
      n114 = while {
        tunnel: w171 -> [w306]
        shift-right: [w267] -> w163
        shift-left: w162 -> [w305]
        tunnel: w180 -> [w302]
        shift-right: [w295] -> w191
        shift-left: w197 -> [w303]
        shift-right: [w294] -> w190
        shift-left: w196 -> [w301]
        shift-right: [w297] -> _
        shift-left: 0 ("binary file indexor in") -> [w300]
        shift-right: [w296] -> _
        shift-left: 0 ("binary file indexor in") -> [w299]
        tunnel: 1000 ("binary file indexor in") -> [w298]
        tunnel: w170 -> [w304]
        tunnel: w173 -> [w273]
        shift-right: [w283] -> _
        shift-left: FALSE -> [w282]
        shift-right: [w279] -> _
        shift-left: 0 -> [w280]
        shift-right: [w278] -> _
        shift-left: w174 -> [w275]
        shift-right: [w277] -> _
        shift-left: w174 -> [w276]
        tunnel: 251 ("y") -> [w274]
        tunnel: w168 -> [w272]
        stop <- w291 stop-if-true
        # "If recording data is on, there should always be elements in the queue, so I shouldn't have to worry about a state where the \"recording data\" is active but there is no data in the queue, if so, then I'll just have to find an alternative to the OR statement"
        n115 = Get Queue Status(queue=w306, error in (no error)=w305) -> (queue out=w288:refnum<queue>, error out=w289:errorcluster, # elements in queue=w284:i32)  [unwired: 1 in, 5 out]
        n116 = local read "Recording Data"() -> (w281:bool)
        n117 = Flush Queue(queue=w288, error in (no error)=w289) -> (remaining elements=w287:T9[], error out=w290:errorcluster)  [unwired: 1 out]
        n118 = Not Equal To 0?(x=w284) -> (x != 0?=w286:bool)
        n119 = And(x=w286, y=w281) -> (x .and. y?=w285:bool)
        n120 = case shown="True" w285 {
          tunnel: w287 -> [_ w398]
          tunnel: w290 -> [w336 w392]
          tunnel: w304 -> [w337 w385]
          tunnel: w303 -> [w344 w397]
          tunnel: w302 -> [w338 w396]
          tunnel: w301 -> [w345 w395]
          tunnel: w300 -> [w343 w394]
          tunnel: w299 -> [w342 w384]
          tunnel: w298 -> [_ w383]
          tunnel: [w343 w391] -> w297
          tunnel: [w342 w390] -> w296
          tunnel: [w344 w387] -> w295
          tunnel: [w345 w386] -> w294
          tunnel: [w335 w377] -> w271
          tunnel: [w334 TRUE] -> w283
          tunnel: w282 -> [w333 _]
          tunnel: w281 -> [w341 _]
          tunnel: w280 -> [w332 w375]
          tunnel: [w331 w374] -> w279
          tunnel: [w330 w381] -> w278
          tunnel: [w329 w378] -> w277
          tunnel: w276 -> [w329 w373]
          tunnel: w275 -> [w330 w372]
          tunnel: w274 -> [_ w366]
          tunnel: w273 -> [w328 _]
          tunnel: w272 -> [w327 _]
          frame False {
            n121 = Not(x=w341) -> (.not. x?=w340:bool)
            n122 = And(x=w340, y=w333) -> (x .and. y?=w339:bool)
            n123 = case shown="True" w339 {
              tunnel: w338 -> [_ w360]
              tunnel: w337 -> [_ w359]
              tunnel: w336 -> [w348 w352]
              tunnel: [w348 w357] -> w335
              tunnel: [w347 FALSE] -> w334
              tunnel: w333 -> [w347 _]
              tunnel: w332 -> [w346 _]
              tunnel: [w346 0] -> w331
              tunnel: w328 -> [_ w350]
              tunnel: w327 -> [_ w349]
              frame False {
              }
              frame True {
                n124 = for {
                  N: w350 -> [_]
                  shift-right: [w363] -> w351
                  shift-left: w352 -> [w364]
                  tunnel: w349 -> [w361] mode=indexing
                  i -> [w362]
                  n125 = property on="Current Measurements Total" class="XYGraph (strict)"(error in=w364, "Active Plot"=w362, "Plot.Plot Color"=w361) -> (error out=w365:errorcluster)  [unwired: 1 in, 1 out]
                  n126 = property on="Voltage Measurements Total" class="XYGraph (strict)"(error in=w365, "Active Plot"=w362, "Plot.Plot Color"=w361) -> (error out=w363:errorcluster)  [unwired: 1 in, 1 out]
                }
                n127 = call "ReadDataFile_V1.vi"("error in (no error)"=w351, "Create CSV files?"=FALSE, "Channel Names Array"=w359, "DataFolder Path"=w360) -> ("error out"=w357:errorcluster, "Current Measurements"=→"Current Measurements Total":cluster{dbl[], dbl[]}[], "Voltage Measurements"=→"Voltage Measurements Total":cluster{dbl[], dbl[]}[])  [unwired: 5 in]
              }
            }
          }
          frame True {
            # "structure where each channel has its own data and supplemental file. Intent for faster data reading speeds in post processing. Probably not since would be i^3, but if we used multiple cores, maybe it would be advantageous"
            n128 = call "FilePathCreation_DCPower_V2.vi"("binary file input reference array 1"=w397, "Channel Name Input array"=w385, "data output directory folder"=w396, "binary file indexor in"=w394, "Reset counter in"=w384, "error in (no error)"=w392, "binary file input reference array 2"=w395, "reset threshold"=w383) -> ("binary file output reference array"=w389:refnum<file>[], "binary file output reference array 2"=w388:refnum<file>[], "binary file indexor out"=w391:i32, "reset counter out"=w390:i32, "error out"=w393:errorcluster)  [unwired: 3 in]
            n129 = for {
              shift-right: [w445] -> w376
              shift-left: w393 -> [w446]
              tunnel: w398 -> [w455]
              tunnel: w388 -> [w452] mode=indexing
              tunnel: w389 -> [w451] mode=indexing
              tunnel: [w450] -> w386 mode=indexing
              tunnel: [w444] -> w387 mode=indexing
              tunnel: [w433] -> w380 mode=indexing
              tunnel: [w432] -> w379 mode=indexing
              i -> [w449]
              n130 = for {
                tunnel: w455 -> [w468] mode=indexing
                tunnel: w449 -> [w465]
                tunnel: [w460] -> w440 mode=concatenating
                tunnel: [w464] -> w454
                tunnel: w452 -> [w463]
                tunnel: w451 -> [w461]
                tunnel: [w461] -> w447
                tunnel: [w463] -> w450
                tunnel: [w462] -> w453 mode=concatenating
                n131 = Unbundle(w468) -> ("Array of fetched data"=w467:dbl[][][], "Channel Names Array"=w466:string[])  [unwired: 3 out]
                n132 = Index Array(array=w466, index=w465) -> (element=w464:string)
                n133 = Index Array(array=w467, index (dim 0)=w465) -> (element=w460:dbl[][])  [unwired: 2 in]
                n134 = Array Size(array=w460) -> (size(s)=w462:i32[])
              }
              n135 = Bundle("Array of fetched data"=w440, w454, w453) -> (w448:T14)  [unwired: 1 in]
              n136 = Index Array(array=w440, index (row)=2) -> (element=w437:dbl[])  [unwired: 1 in]
              n137 = Index Array(array=w440, index (row)=1) -> (element=w438:dbl[])  [unwired: 1 in]
              n138 = Index Array(array=w440, index (row)=0) -> (element=w439:dbl[])  [unwired: 1 in]
              n139 = call "DataFileNode_Entry_V4.vi"("error in (no error)"=w446, "Queued Elements"=w448, "Byte Stream File in"=w447) -> ("error out"=w445:errorcluster, "Byte Stream File out"=w444:refnum<file>)  [unwired: 7 in]
              n140 = for {
                tunnel: [w457] -> w436 mode=indexing if=w456
                tunnel: w439 -> [w457] mode=indexing
                tunnel: [w459] -> w434 mode=indexing if=w456
                tunnel: w438 -> [w459] mode=indexing
                tunnel: [w458] -> w435 mode=indexing if=w456
                tunnel: w437 -> [w458] mode=indexing
                n141 = Not Equal To 0?(x=w457) -> (x != 0?=w456:bool)
              }
              n142 = Bundle(w436, w434) -> (w433:cluster{dbl[], dbl[]})  [unwired: 1 in]
              n143 = Bundle(w436, w435) -> (w432:cluster{dbl[], dbl[]})  [unwired: 1 in]
            }
            n144 = Greater?(x=w375, y=w366) -> (0:w368:bool)
            n145 = Array Size(array=w372) -> (size(s)=w371:i32)
            n146 = Equal?(x=w371, y=0) -> (x = y?=w369:bool)
            n147 = Or(x=w368, y=w369) -> (x .or. y?=w367:bool)
            n148 = case shown="False" w367 {
              tunnel: [w404 w428] -> w381
              tunnel: w372 -> [w408 _]
              tunnel: w380 -> [w407 w428]
              tunnel: w373 -> [w406 _]
              tunnel: w379 -> [w405 w429]
              tunnel: [w403 w429] -> w378
              tunnel: [w402 w431] -> w377
              tunnel: w376 -> [w401 w431]
              tunnel: w375 -> [w400 _]
              tunnel: [w399 0] -> w374
              frame False {
                n149 = for {
                  tunnel: w408 -> [w427] mode=indexing
                  tunnel: w407 -> [w424] mode=indexing
                  tunnel: w406 -> [w421] mode=indexing
                  tunnel: w405 -> [w420] mode=indexing
                  tunnel: [w411] -> w404 mode=indexing
                  tunnel: [w410] -> w403 mode=indexing
                  shift-right: [w409] -> w402
                  shift-left: w401 -> [w409]
                  n150 = Unbundle(w427) -> (w426:dbl[], w425:dbl[])
                  n151 = Unbundle(w424) -> (w423:dbl[], w422:dbl[])
                  n152 = Unbundle(w421) -> (w419:dbl[], w418:dbl[])
                  n153 = Unbundle(w420) -> (w417:dbl[], w416:dbl[])
                  n154 = Insert Into Array(array=w419, new element=w417) -> (w414:dbl[])  [unwired: 1 in]
                  n155 = Insert Into Array(array=w426, new element=w423) -> (w412:dbl[])  [unwired: 1 in]
                  n156 = Insert Into Array(array=w418, new element=w416) -> (w415:dbl[])  [unwired: 1 in]
                  n157 = Insert Into Array(array=w425, new element=w422) -> (w413:dbl[])  [unwired: 1 in]
                  n158 = Bundle(w414, w415) -> (w410:cluster{dbl[], dbl[]})  [unwired: 1 in]
                  n159 = Bundle(w412, w413) -> (w411:cluster{dbl[], dbl[]})  [unwired: 1 in]
                }
                n160 = Increment(x=w400) -> (x+1=w399:i32)
              }
              frame True {
              }
            }
            "Voltage Measurements Live" <- w381
            "Current Measurements Live" <- w378
          }
        }
        n161 = Equal To 0?(x=w284) -> (x = 0?=w292:bool)
        n162 = case shown="True" "Live Measurement Range Update" {
          tunnel: w271 -> [w317 w326]
          tunnel: [w317 w325] -> w268
          frame False {
          }
          frame True {
            (unwired) 0.001 ("Delay Time (s)")
            n163 = property on="Voltage Measurements Live" class="XYGraph (strict)"(error in=w326, "YScale.Maximum"="Live Voltage Y Max", "YScale.Minimum"="Live Voltage Y Min") -> (error out=w319:errorcluster)  [unwired: 1 in, 1 out]
            n164 = property on="Current Measurements Live" class="XYGraph (strict)"(error in=w319, "ActXScl"=0 ("Active X Scale")) -> (error out=w318:errorcluster)  [unwired: 1 in, 1 out]
            n165 = property on="Current Measurements Live" class="XYGraph (strict)"(error in=w318, "YScale.Maximum"="Live Current Y Max", "YScale.Minimum"="Live Current Y Min") -> (error out=w325:errorcluster)  [unwired: 1 in, 1 out]
          }
        }
        n166 = local read "Exiting"() -> (w293:bool)
        n167 = And(x=w292, y=w293) -> (x .and. y?=w291:bool)
        n168 = case shown="True" "Total Measurement Range Update" {
          tunnel: w268 -> [w307 w316]
          tunnel: [w307 w314] -> w267
          frame False {
          }
          frame True {
            n169 = property on="Voltage Measurements Total" class="XYGraph (strict)"(error in=w316, "YScale.Maximum"="Total Voltage Y Max", "YScale.Minimum"="Total Voltage Y Min", "XScale.Maximum"="Total Time X Max", "XScale.Minimum"="Total Time X Min") -> (error out=w315:errorcluster)  [unwired: 1 in, 1 out]
            n170 = property on="Current Measurements Total" class="XYGraph (strict)"(error in=w315, "YScale.Maximum"="Total Current Y Max", "YScale.Minimum"="Total Current Y Min", "XScale.Maximum"="Total Time X Max", "XScale.Minimum"="Total Time X Min") -> (error out=w314:errorcluster)  [unwired: 1 in, 1 out]
          }
        }
      }
      n171 = Merge Errors(w163, w165) -> (w164:errorcluster)
      n172 = for {
        tunnel: w191 -> [w611] mode=indexing
        tunnel: w190 -> [w609] mode=indexing
        shift-right: [w607] -> w189
        shift-left: w164 -> [w610]
        n173 = Close File(refnum=w611, error in=w610) -> (error out=w608:errorcluster)  [unwired: 1 out]
        n174 = Close File(refnum=w609, error in=w608) -> (error out=w607:errorcluster)  [unwired: 1 out]
      }
    }
    frame Disabled {
      n175 = for {
        tunnel: w613 -> [w639] mode=indexing
        shift-right: [w635] -> w614
        shift-left: w615 -> [w637]
        w633 = 388 items=["Start"=482, "Trigger"=483, "Pretrigger"=477, "Now"=481, "Read Pointer"=388] ("Fetch:Fetch Relative To")
        n176 = Unbundle By Name(w639) -> ("instrument handle out"=w638:refnum<k15>)
        n177 = call <instrlib>:"niScope Initiate Acquisition.vi"("instrument handle"=w638, "error in"=w637) -> ("instrument handle out"=w634:refnum<k15>, "error out"=w636:errorcluster)  [unwired: 12 in]
        n178 = property class="niScope"(reference=w634, error in=w636, "Fetch Relative To"=w633) -> (error out=w635:errorcluster)  [unwired: 1 out]
      }
      n179 = while {
        tunnel: w613 -> [w624]
        shift-right: [w620] -> w612
        shift-left: w614 -> [w623]
        stop <- "stop" stop-if-true
        n180 = for {
          tunnel: w624 -> [w632] mode=indexing
          shift-right: [w627] -> w620
          shift-left: w623 -> [w631]
          tunnel: [w626] -> w622 mode=indexing
          n181 = Unbundle By Name(w632) -> ("instrument handle out"=w630:refnum<k15>, "channel names list"=w629:string)
          n182 = call-poly <instrlib>:"niScope Fetch (poly).vi"("timeout"=0.0, "error in"=w631, "numSamples"=-1, "channels"=w629, "instrument handle"=w630) -> ("error out"=w627:errorcluster, "wfm"=w626:i16[][])  [unwired: 3 in, 2 out]
        }
        "wfm 2" <- w622
      }
    }
  }
  n183 = Merge Errors(w42, w40) -> (w39:errorcluster)
  n184 = Unbundle(w38) -> ("created path"=w14:path)  [unwired: 2 out]
  n185 = case shown="True" w30 {
    selector: w30 -> [w646 w786]
    tunnel: w39 -> [w641 w792]
    tunnel: [w650 w724] -> w9
    tunnel: w2 -> [w650 w791]
    tunnel: [w649 w726] -> w37
    tunnel: w36 -> [w649 w790]
    tunnel: [w648 w712] -> w35
    tunnel: w34 -> [w648 w789]
    tunnel: [w647 w729] -> w33
    tunnel: w32 -> [w647 w788]
    tunnel: [w642 w731] -> w6
    tunnel: w31 -> [w642 w787]
    tunnel: [w646 w786] -> w29
    tunnel: [string[][] [] ("DCPowerInfoArray") w722] -> w28
    tunnel: w14 -> [_ w657]
    tunnel: [string[][] [] ("DCPowerInfoArray") w720] -> w10
    tunnel: [string[][] [] ("DCPowerInfoArray") w714] -> w21
    tunnel: [w640 w659] -> w13
    tunnel: w12 -> [_ w658]
    frame False {
      (unwired) string[][][] []
      n186 = for {
        tunnel: w642 -> [w653] mode=indexing
        shift-right: [w654] -> w640
        shift-left: w641 -> [w655]
        n187 = Unbundle(w653) -> ("IVI Refnum out"=w652:refnum<k15>, "Active Channel Numbers String List"=w651:string)  [unwired: 6 out]
        n188 = call <instrlib>:"niDCPower Abort With Channels.vi"("error in (no error)"=w655, "channel name"=w651, "instrument handle"=w652) -> ("error out"=w654:errorcluster)  [unwired: 7 in, 1 out]
      }
    }
    frame True {
      # "This will be indexed eventually"
      n189 = for {
        shift-right: [w886] -> w656
        shift-left: w792 -> [w897]
        tunnel: w787 -> [w884] mode=indexing
        shift-right: [w896] -> w762
        shift-left: w791 -> [w896]
        shift-right: [w895] -> w761
        shift-left: w790 -> [w895]
        shift-right: [w894] -> w760
        shift-left: w789 -> [w894]
        shift-right: [w893] -> w759
        shift-left: w788 -> [w893]
        shift-right: [w892] -> w758
        shift-left: w787 -> [w892]
        shift-right: [w890] -> w763
        shift-left: string[][] [] ("DCPowerInfoArray") -> [w891]
        # "This puts all the instruments together in one output"
        n190 = Unbundle(w884) -> ("IVI Refnum out"=w899:refnum<k15>, "Active Channel Numbers String List"=w898:string)  [unwired: 6 out]
        n191 = call <instrlib>:"niDCPower Abort With Channels.vi"("error in (no error)"=w897, "channel name"=w898, "instrument handle"=w899) -> ("error out"=w887:errorcluster)  [unwired: 7 in, 1 out]
        n192 = call "DCPower_ParameterCreation.vi"("error in"=w887, "Precision"="8", "DCPowerInformationByInstrument"=w884) -> ("error out"=w886:errorcluster, "DCPowerInfoArray"=w885:string[][])
        n193 = Insert Into Array(array=w891, index (col)=0 ("disabled index (col)"), new element=w885) -> (w890:string[][])  [unwired: 1 in]
      }
      n194 = Concatenate Strings("Channel Name " ("string")) -> (w775:string)
      n195 = Concatenate Strings("Voltage (V) " ("string")) -> (w777:string)
      n196 = Concatenate Strings("Measure Record delta Time (s) " ("string")) -> (w779:string)
      n197 = Concatenate Strings("Instrument Name " ("string")) -> (w774:string)
      n198 = Concatenate Strings("Instrument Channel Number " ("string")) -> (w776:string)
      n199 = Concatenate Strings("Current Limit (A) " ("string")) -> (w778:string)
      n200 = Build Array(w774, w775, w776, w777, w778, w779) -> (w767:string[])
      n201 = Build Path(base path=w657, name or relative path="DCPOW_Params.csv") -> (appended path=w782:path)
      n202 = Insert Into Array(array=w763, index (col)=0 ("disabled index (col)"), new element=w767) -> (w766:string[][])  [unwired: 1 in]
      n203 = call-poly <vilib>:"Write Delimited Spreadsheet.vi"("file path (dialog if empty)"=w782, "format (%s)"="%s" ("format (%.3f)"), "2D data"=w766, "error in (no error)"=w656, "transpose? (no:F)"=TRUE, "delimiter (\\t)"="," ("delimiter (\\t)")) -> ("error out"=w764:errorcluster)  [unwired: 8 in, 1 out]
      n204 = for {
        shift-right: [w878] -> w744
        shift-left: w764 -> [w878]
        shift-right: [w873] -> w732
        shift-left: w758 -> [w873]
        shift-right: [w874] -> w730
        shift-left: w759 -> [w874]
        shift-right: [w875] -> w728
        shift-left: w760 -> [w875]
        shift-right: [w876] -> w727
        shift-left: w761 -> [w876]
        shift-right: [w877] -> w723
        shift-left: w763 -> [w877]
        tunnel: w762 -> [w872] mode=indexing
        tunnel: [w872] -> w725 mode=indexing
        shift-right: [w841] -> w721
        shift-left: string[][] [] ("DCPowerInfoArray") -> [w847]
        n205 = Unbundle(w872) -> ("instrument handle out"=w871:refnum<k15>, w844:string[], w845:string[], "vertical range"=w866:dbl, "vertical coupling"=w860:T1, "Channel 0 50 ohms?"=w865:bool, "50 ohm vertical range (V)"=w864:dbl, "min record length"=w859:i32, "Actual Sample Rate"=w858:dbl)  [unwired: 1 out]
        n206 = Array Size(array=w844) -> (size(s)=w867:i32)
        n207 = Initialize Array(w866, w867) -> (w863:dbl[])
        n208 = Decimal String To Number(string="8") -> (number=w842:i32)  [unwired: 2 in, 1 out]
        n209 = case shown="True" w865 {
          tunnel: w864 -> [_ w881]
          tunnel: w863 -> [w879 w883]
          tunnel: [w879 w880] -> w862
          frame False {
          }
          frame True {
            n210 = Replace Array Subset(array=w883, new element=w881, index=0) -> (w880:dbl[])
          }
        }
        n211 = Number To Fractional String(number=w858, precision (6)=w842) -> (F-format string=w852:string)  [unwired: 2 in]
        n212 = Number To Decimal String(number=w859) -> (decimal integer string=w853:string)  [unwired: 1 in]
        n213 = Concatenate Strings(w871) -> (w869:string)
        n214 = Number To Fractional String(number=w862, precision (6)=w842) -> (F-format string=w861:string[])  [unwired: 2 in]
        n215 = Number To Decimal String(number=w860) -> (decimal integer string=w854:string)  [unwired: 1 in]
        n216 = Array Size(array=w844) -> (size(s)=w870:i32)
        n217 = Initialize Array(w869, w870) -> (w868:string[])
        n218 = Array Size(array=w844) -> (size(s)=w857:i32)
        n219 = Array Size(array=w844) -> (size(s)=w855:i32)
        n220 = Array Size(array=w844) -> (size(s)=w856:i32)
        n221 = Initialize Array(w854, w857) -> (w851:string[])
        n222 = Initialize Array(w852, w855) -> (w849:string[])
        n223 = Initialize Array(w853, w856) -> (w850:string[])
        n224 = Build Array(w868, w845, w844, w861, w851, w850, w849) -> (w846:string[][])
        n225 = Insert Into Array(array=w847, index (col)=0 ("disabled index (col)"), new element=w846) -> (w841:string[][])  [unwired: 1 in]
      }
      n226 = Build Array("Instrument Name " ("string"), "Channel Name" ("element"), "Instrument Channel Number" ("element"), "Vertical Range (V)" ("element"), "Vertical Coupling" ("element"), "Min Record Length" ("element"), "Actual Sample Rate" ("element")) -> (w748:string[])
      n227 = Insert Into Array(array=w721, index (col)=0 ("disabled index (col)"), new element=w748) -> (w741:string[][])  [unwired: 1 in]
      n228 = Build Path(base path=w657, name or relative path="Oscilloscope_Params.csv") -> (appended path=w746:path)
      n229 = call-poly <vilib>:"Write Delimited Spreadsheet.vi"("file path (dialog if empty)"=w746, "format (%s)"="%s" ("format (%.3f)"), "2D data"=w741, "error in (no error)"=w744, "transpose? (no:F)"=TRUE, "delimiter (\\t)"="," ("delimiter (\\t)")) -> ("error out"=w739:errorcluster)  [unwired: 8 in, 1 out]
      n230 = for {
        shift-right: [w823] -> w737
        shift-left: string[][] [] ("DCPowerInfoArray") -> [w824]
        tunnel: w727 -> [w839] mode=indexing
        shift-right: [w808] -> w713
        shift-left: w739 -> [w815]
        shift-right: [w816] -> w720
        shift-left: w721 -> [w816]
        shift-right: [w817] -> w722
        shift-left: w723 -> [w817]
        shift-right: [w818] -> w724
        shift-left: w725 -> [w818]
        shift-right: [w819] -> w726
        shift-left: w727 -> [w819]
        shift-right: [w820] -> w712
        shift-left: w728 -> [w820]
        shift-right: [w821] -> w729
        shift-left: w730 -> [w821]
        shift-right: [w822] -> w731
        shift-left: w732 -> [w822]
        n231 = Unbundle(w839) -> ("VISA resource name"=w838:refnum<visa-resource-name>, "Frequency (GHz) Output"=w832:dbl, "Power (dBm) Output"=w829:dbl)  [unwired: 2 out]
        n232 = Decimal String To Number(string="8") -> (number=w827:i32)  [unwired: 2 in, 1 out]
        n233 = VISA Write(VISA resource name=w838, write buffer="*IDN?", error in (no error)=w815) -> (VISA resource name out=w834:refnum<visa-resource-name>, return count=w836:u32, error out=w840:errorcluster)
        n234 = Number To Fractional String(number=w829, precision (6)=w827) -> (F-format string=w830:string)  [unwired: 2 in]
        n235 = Add(x=w836, y=u32 10) -> (x+y=w833:u32)
        n236 = Number To Fractional String(number=w832, precision (6)=w827) -> (F-format string=w831:string)  [unwired: 2 in]
        n237 = VISA Read(VISA resource name=w834, byte count=w833, error in (no error)=w840) -> (read buffer=w814:string, error out=w809:errorcluster)  [unwired: 2 out]
        n238 = Search and Replace String(replace all?=TRUE ("replace all? (F)"), input string=w814, search string=",", replace string="_" ("replace string (\"\")"), error in=w809) -> (result string=w811:string, error out=w808:errorcluster)  [unwired: 3 in, 2 out]
        n239 = Build Array(w811, w831, w830) -> (w826:string[])
        n240 = Insert Into Array(array=w824, index (col)=0 ("index (row)"), new element=w826) -> (w823:string[][])  [unwired: 1 in]
      }
      n241 = Build Array("Instrument Name", "Frequency (GHz)" ("element"), "Power (dBm)" ("element")) -> (w733:string[])
      n242 = Build Path(base path=w657, name or relative path="RFSource_Params.csv") -> (appended path=w718:path)
      n243 = Insert Into Array(array=w737, index (col)=0 ("disabled index (col)"), new element=w733) -> (w714:string[][])  [unwired: 1 in]
      n244 = call-poly <vilib>:"Write Delimited Spreadsheet.vi"("file path (dialog if empty)"=w718, "format (%s)"="%s" ("format (%.3f)"), "2D data"=w714, "error in (no error)"=w713, "transpose? (no:F)"=TRUE, "delimiter (\\t)"="," ("delimiter (\\t)")) -> ("error out"=w693:errorcluster)  [unwired: 8 in, 1 out]
      n245 = Strip Path(path=w657) -> (name=w711:string)  [unwired: 1 out]
      n246 = Unbundle(w712) -> ("DUT"=w710:string, "Ion (ex Kr)"=w709:string, "Board Number"=w708:string, "Effective LET"=w707:string, "Test Type"=w706:T16)  [unwired: 1 out]
      n247 = case shown="\"Single Event Latchup\", Default" w706 {
        tunnel: ["Single Event Latchup (SEL)" "Single Event Transient (SET)"] -> w705
        frame "Single Event Latchup", Default {
        }
        frame "Single Event Transient" {
        }
      }
      n248 = Build Array("Run Number" ("name"), "DUT" ("element"), "Ion" ("element"), "Board Number" ("element"), "Effective LET" ("element"), "Test Type" ("element")) -> (w704:string[])
      n249 = Build Array(w711, w710, w709, w708, w707, w705) -> (w703:string[])
      n250 = Build Array(w704, w703) -> (w692:string[][])
      n251 = Build Path(base path=w657, name or relative path="RunData_Params.csv") -> (appended path=w698:path)
      n252 = call-poly <vilib>:"Write Delimited Spreadsheet.vi"("file path (dialog if empty)"=w698, "format (%s)"="%s" ("format (%.3f)"), "2D data"=w692, "error in (no error)"=w693, "transpose? (no:F)"=TRUE, "delimiter (\\t)"="," ("delimiter (\\t)")) -> ()  [unwired: 8 in, 2 out]
      n253 = List Folder(path=w657, pattern="*NULL.txt") -> (path out=w676:path, filenames=w677:string[], error out=w678:errorcluster)  [unwired: 2 in, 1 out]
      n254 = for {
        tunnel: [w793] -> w688
        tunnel: w676 -> [w793]
        tunnel: w677 -> [w795] mode=indexing
        shift-right: [w796] -> w679
        shift-left: w678 -> [w797]
        n255 = Build Path(base path=w793, name or relative path=w795) -> (appended path=w794:path)
        n256 = Delete(path (use dialog)=w794, error in=w797) -> (error out=w796:errorcluster)  [unwired: 3 in, 2 out]
      }
      n257 = Get Date/Time String(date format (0)=enum16{"short", "long", "abbreviated"}."short", seconds (now)=w658, want seconds? (F)=TRUE) -> (date string=w682:string, time string=w681:string)
      n258 = Concatenate Strings(w682, "_" ("string"), w681) -> (w683:string)
      n259 = Strip Path(path=w688) -> (name=w674:string)  [unwired: 1 out]
      n260 = Build Path(base path=w688, name or relative path="BeginRecordTimeStamp.txt") -> (appended path=w689:path)
      n261 = Concatenate Strings(w674, "_DCPOWER_COPYFOLDER" ("name or relative path")) -> (w675:string)
      n262 = Open/Create/Replace File(file path (use dialog)=w689, error in=w679, operation (0:open)=T15."open or create", access (0:read/write)=enum16{"read/write", "read-only", "write-only"}."read/write") -> (refnum out=w684:refnum<file>, error out=w680:errorcluster)  [unwired: 2 in, 1 out]
      n263 = Build Path(base path=w688, name or relative path=w675) -> (appended path=w668:path)
      n264 = Write to Text File(file (use dialog)=w684, text=w683, error in=w680) -> (refnum out=w686:refnum<file>, error out=w685:errorcluster)  [unwired: 1 in, 1 out]
      n265 = Close File(refnum=w686, error in=w685) -> (error out=w687:errorcluster)  [unwired: 1 out]
      n266 = Create Folder(path (use dialog)=w668, error in=w687) -> (created path=w672:path, error out=w669:errorcluster)  [unwired: 1 in, 1 out]
      n267 = List Folder(path=w688, error in=w669) -> (path out=w670:path, filenames=w671:string[], error out=w673:errorcluster)  [unwired: 2 in, 1 out]
      n268 = for {
        tunnel: w670 -> [w803]
        tunnel: w671 -> [w802] mode=indexing
        tunnel: w672 -> [w798]
        shift-right: [w805] -> w659
        shift-left: w673 -> [w799]
        tunnel: [w798] -> _
        n269 = Build Path(base path=w803, name or relative path=w802) -> (appended path=w800:path)
        n270 = Build Path(base path=w798, name or relative path=w802) -> (appended path=w801:path)
        n271 = Copy(8:w799, 9:TRUE ("overwrite (F)"), 10:w801, 11:w800) -> (0:w805:errorcluster)  [unwired: 1 in, 2 out]
      }
    }
  }
  "VISAPowerInfoInputOutput" <- w33
  "Run Data SubPanel Output" <- w35
  "Data Was Collected?" <- w29
  "DCPowerInfoArray" <- w28
  "OscilloscopeInfoArray" <- w10
  "RFSourceInfoArray" <- w21
  "RF Subpanel Output" <- w37
  "error out" <- w13
  "Oscilloscope Info Array" <- w9
  "DCPowerInformationClusterArray_Output" <- w6
